vi "Run Process.vi"(8 "error in (no error)":errorcluster, 9 "Processes":cluster{"VI":refnum<vi>, "Parameters":variant}[](array[cluster]), 11 "Async in":refnum<class "VS Inline Async API.lvclass">) -> (0 "error out":errorcluster, 3 "Async out":refnum<class "VS Inline Async API.lvclass">)   [LabVIEW 2015, in "VS Inline Async API.lvlib" / "VS Inline Async API.lvclass"]
uses:
  VS Inline Async API.lvclass
  VS Inline Async API.lvclass/VS Inline Async API.ctl
  Process/Process.lvclass
  Process/Process.lvclass/Process.ctl
  Process/Data Member Access/Write Name.vi
  Process/Data Member Access/Write Process.Stop.vi
  Process/Data Member Access/Write Process.Trigger.vi
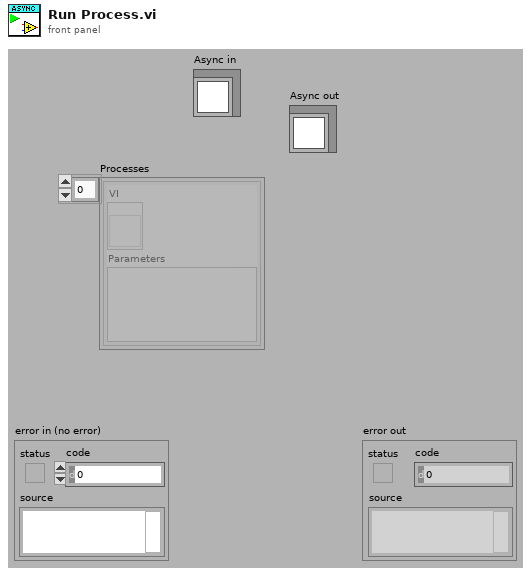
[diagram p1: front panel]
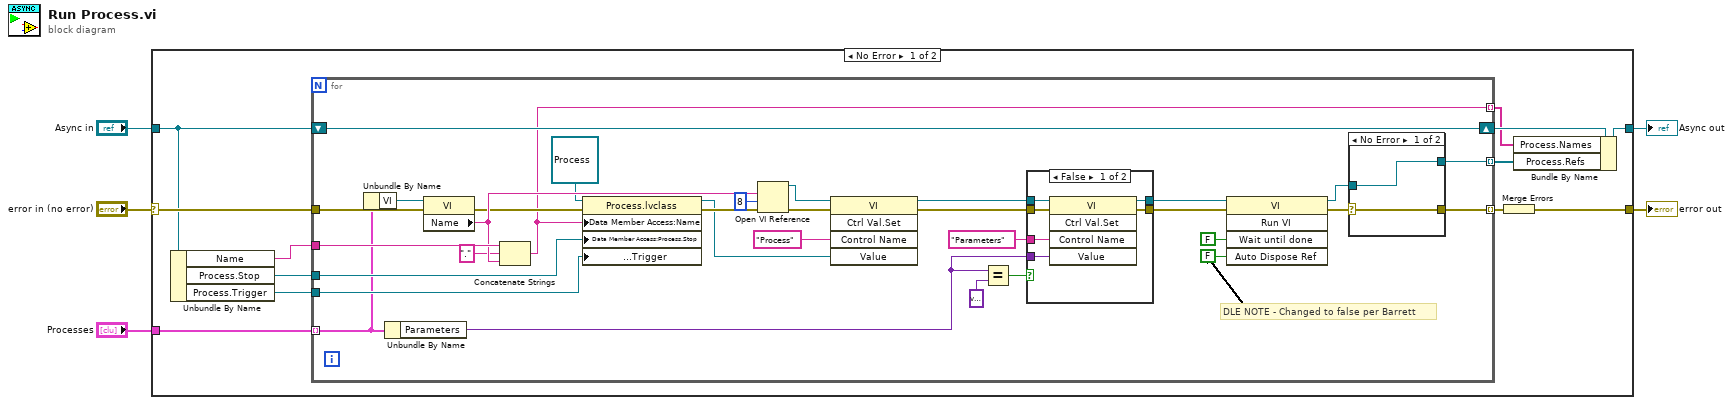
[diagram p0: block diagram]
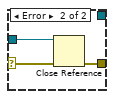
[diagram p3: hidden frame]
diagram:
  n1 = case shown="No Error" "error in (no error)" {
    selector: "error in (no error)" -> [w16 w64]
    tunnel: [w14 w64] -> w5
    tunnel: "Processes" -> [w15 _]
    tunnel: "Async in" -> [w10 w63]
    tunnel: [w11 w63] -> w1
    frame No Error {
      n2 = Unbundle By Name(w10) -> ("Name"=w9:string, "Process.Stop"=w8:refnum<data-value>, "Process.Trigger"=w7:refnum<notifier>)
      n3 = for {
        tunnel: [w49] -> w17 mode=indexing
        tunnel: [w48] -> w13 mode=indexing
        tunnel: w16 -> [w35]
        tunnel: w15 -> [w22] mode=indexing
        shift-right: [w34] -> w12
        shift-left: w10 -> [w34]
        tunnel: w9 -> [w33]
        tunnel: w8 -> [w27]
        tunnel: w7 -> [w26]
        tunnel: [w24] -> w6 mode=indexing
        # "DLE NOTE - Changed to false per Barrett"
        n4 = Unbundle By Name(w22) -> ("VI"=w23:refnum<vi>)
        n5 = Unbundle By Name(w22) -> ("Parameters"=w21:variant)
        n6 = property class="VI"(reference=w23, error in=w35) -> (error out=w29:errorcluster, "Name"=w32:string)  [unwired: 1 out]
        n7 = Concatenate Strings(w33, "." ("string"), w32) -> (w24:string)
        n8 = property class="Process.lvclass"(reference=refnum<class "Process.lvclass"> refnum ("VS Inline Async API.lvlib:Process.lvclass"), error in=w29, "Data Member Access:Name"=w24, "Data Member Access:Process.Stop"=w27, "Data Member Access:Process.Trigger"=w26) -> (reference out=w25:refnum<class "Process.lvclass">, error out=w28:errorcluster)
        n9 = Open VI Reference(vi path=w32, options=8, error in (no error)=w28) -> (vi reference=w36:refnum<vi>, error out=w39:errorcluster)  [unwired: 3 out]
        n10 = invoke class="VI" method="Ctrl Val.Set"(reference=w36, error in=w39, "Control Name"="Process", "Value"=w25) -> (reference out=w37:refnum<vi>, error out=w38:errorcluster)  [unwired: 1 in, 3 out]
        n11 = Equal?(x=w21, y=variant) -> (x = y?=w19:bool)
        n12 = case shown="False" w19 {
          tunnel: [w55 w57] -> w43
          tunnel: [w54 w56] -> w42
          tunnel: w38 -> [w53 w57]
          tunnel: w37 -> [w52 w56]
          tunnel: "Parameters" ("Control Name") -> [w51 _]
          tunnel: w21 -> [w50 _]
          frame False {
            n13 = invoke class="VI" method="Ctrl Val.Set"(reference=w52, error in=w53, "Control Name"=w51, "Value"=w50) -> (reference out=w54:refnum<vi>, error out=w55:errorcluster)  [unwired: 1 in, 3 out]
          }
          frame True {
          }
        }
        n14 = invoke class="VI" method="Run VI"(reference=w42, error in=w43, "Wait until done"=FALSE ("Wait Until Done"), "Auto Dispose Ref"=FALSE ("Auto Dispose Reference")) -> (reference out=w44:refnum<vi>, error out=w45:errorcluster)  [unwired: 1 in, 3 out]
        n15 = case shown="No Error" w45 {
          selector: w45 -> [w59 w62]
          tunnel: w44 -> [w58 w61]
          tunnel: [w59 w60] -> w49
          tunnel: [w58 _] -> w48
          frame No Error {
          }
          frame Error {
            n16 = Close Reference(reference=w61, error in (no error)=w62) -> (error out=w60:errorcluster)
          }
        }
      }
      n17 = Merge Errors(w17) -> (w14:errorcluster)
      n18 = Bundle By Name(cluster=w12, "Process.Names"=w6, "Process.Refs"=w13) -> (w11:refnum<class "VS Inline Async API.lvclass">)
    }
    frame Error {
    }
  }
  "error out" <- w5
  "Async out" <- w1
